vi "Get Contents.vi"(8 "error in (no error)":errorcluster caption="错误输入（无错误）", 11 "Dictionary In":refnum<class "Dictionary.lvclass"> caption="DNL_LabVIEW Object in") -> (0 "error out":errorcluster caption="错误输出", 1 "Values Array":string[](array[string]), 2 "Keys Array":string[](array[string]), 3 "Dictionary Out":refnum<class "Dictionary.lvclass"> caption="DNL_LabVIEW Object out")   [LabVIEW 2012, in "Dictionary.lvclass"]
uses:
  Dictionary.lvclass
  Dictionary.lvclass/Dictionary.ctl
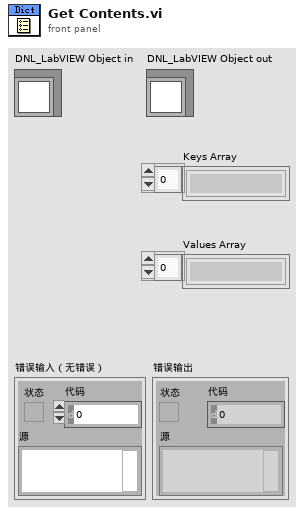
[diagram p1: front panel]
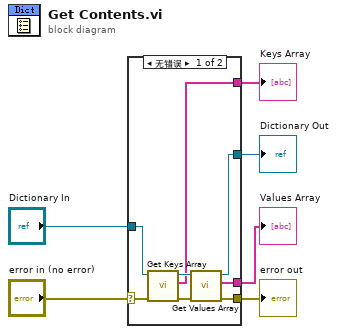
[diagram p0: block diagram]
diagram:
  n1 = case shown="无错误" "error in (no error)" {
    selector: "error in (no error)" -> [w11 w16]
    tunnel: [w9 w16] -> w5
    tunnel: [w12 w15] -> w3
    tunnel: "Dictionary In" -> [w14 w15]
    tunnel: [w8 _] -> w2
    tunnel: [w7 _] -> w1
    frame No Error {
      n2 = call "Get Keys Array.vi"("error in"=w11, "Dictionary in"=w14) -> ("error out"=w10:errorcluster, "Keys Array"=w8:string[], "Dictionary out"=w13:refnum<class "Dictionary.lvclass">)  [unwired: 7 in]
      n3 = call "Get Values Array.vi"("error in"=w10, "Dictionary in"=w13) -> ("error out"=w9:errorcluster, "Values Array"=w7:string[], "Dictionary out"=w12:refnum<class "Dictionary.lvclass">)  [unwired: 7 in]
    }
    frame Error {
    }
  }
  "error out" <- w5
  "Dictionary Out" <- w3
  "Keys Array" <- w2
  "Values Array" <- w1
